vi "stepper graphics controller.vi"(4 "cursor index":i32, 6 "stepper motor state":T3, 7 "stepper graphics action":T1=enum."void", 8 "stepper graphics internal state":T2, 10 "value":dbl=1.0 format="%#_13g") -> (0 "stepper graphics internal state OUT":T2, 1 "current pos":dbl, 2 "set pos":dbl)   [LabVIEW 2018]
uses:
  stepper motor state.ctl
  stepper graphics internal state.ctl
  stepper graphics action.ctl
  2Dwindow.ctl
  slider action.ctl
  cursor action.ctl
  generate linear region.vi
  generate linear region --complex -- win cen.vi
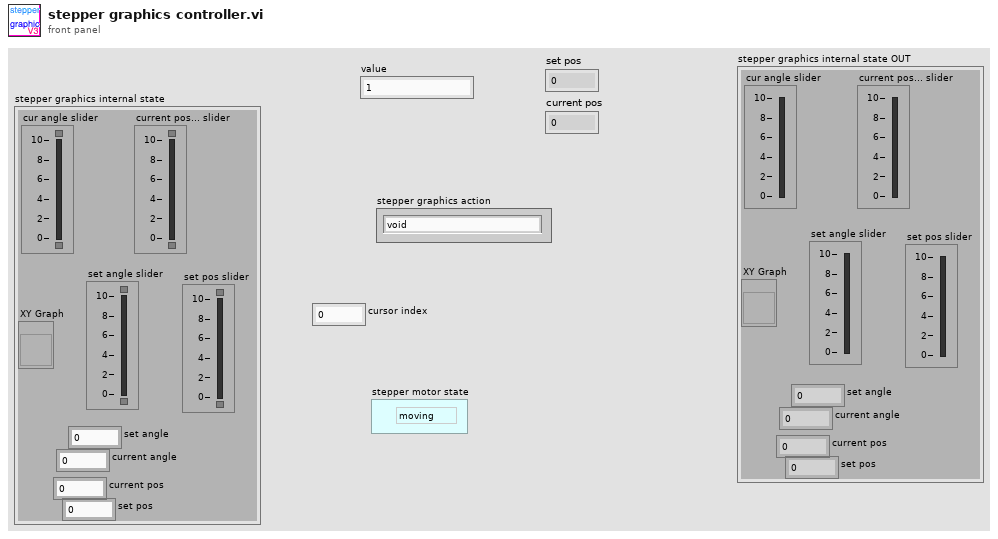
[diagram p1: front panel]
types:
  T1 = typedef "stepper graphics action.ctl" = enum16{"--update circle", "set step slider moves", "cursor moves", "current pos changed", "init", "void", "--draw current lie", "--draw set line", "--move current step slider", "--move set step slider", "--draw limit lines", "check", "--move set angle slider", "--move current angle slider", "set angle slider moves", "--move center cursor", "set set step", "set current step", "read", "--move limit-cursors", "cursor release"}
  T2 = typedef "stepper graphics internal state.ctl" = cluster{"set pos slider":refnum<vi>, "cur angle slider":refnum<vi>, "XY Graph":refnum<vi>, "set angle":dbl, "current angle":dbl, "set angle slider":refnum<vi>, "current pos... slider":refnum<vi>, "current pos":dbl, "set pos":dbl}
  T3 = typedef "stepper motor state.ctl" = enum16{"moving", "stopped"}
  T4 = typedef "2Dwindow.ctl" = cluster{"window y":dbl, "center x":dbl, "center y":dbl, "window x":dbl}
  T5 = typedef "slider action.ctl" = enum16{"check", "copy range", "set from value", "set from ratio", "set from slider", "read using other slider", "set lower limit", "set upper limit", "set lower from slider", "set upper from slider"}
  T6 = typedef "cursor action.ctl" = enum16{"range", "read", "write", "check", "zoom out", "smart zoom out", "zoom to aspect ratio 1", "zoom to win", "zoom out 20%", "zoom in 20%", "-empty", "smart zoom out&aspect", "move range left 20%", "move range right 20%", "move range up 20%", "move range down 20%", "zoom to X win", "zoom to Y win", "zoom out X", "zoom out Y", "zoom in X", "zoom in Y", "check plot scale"}
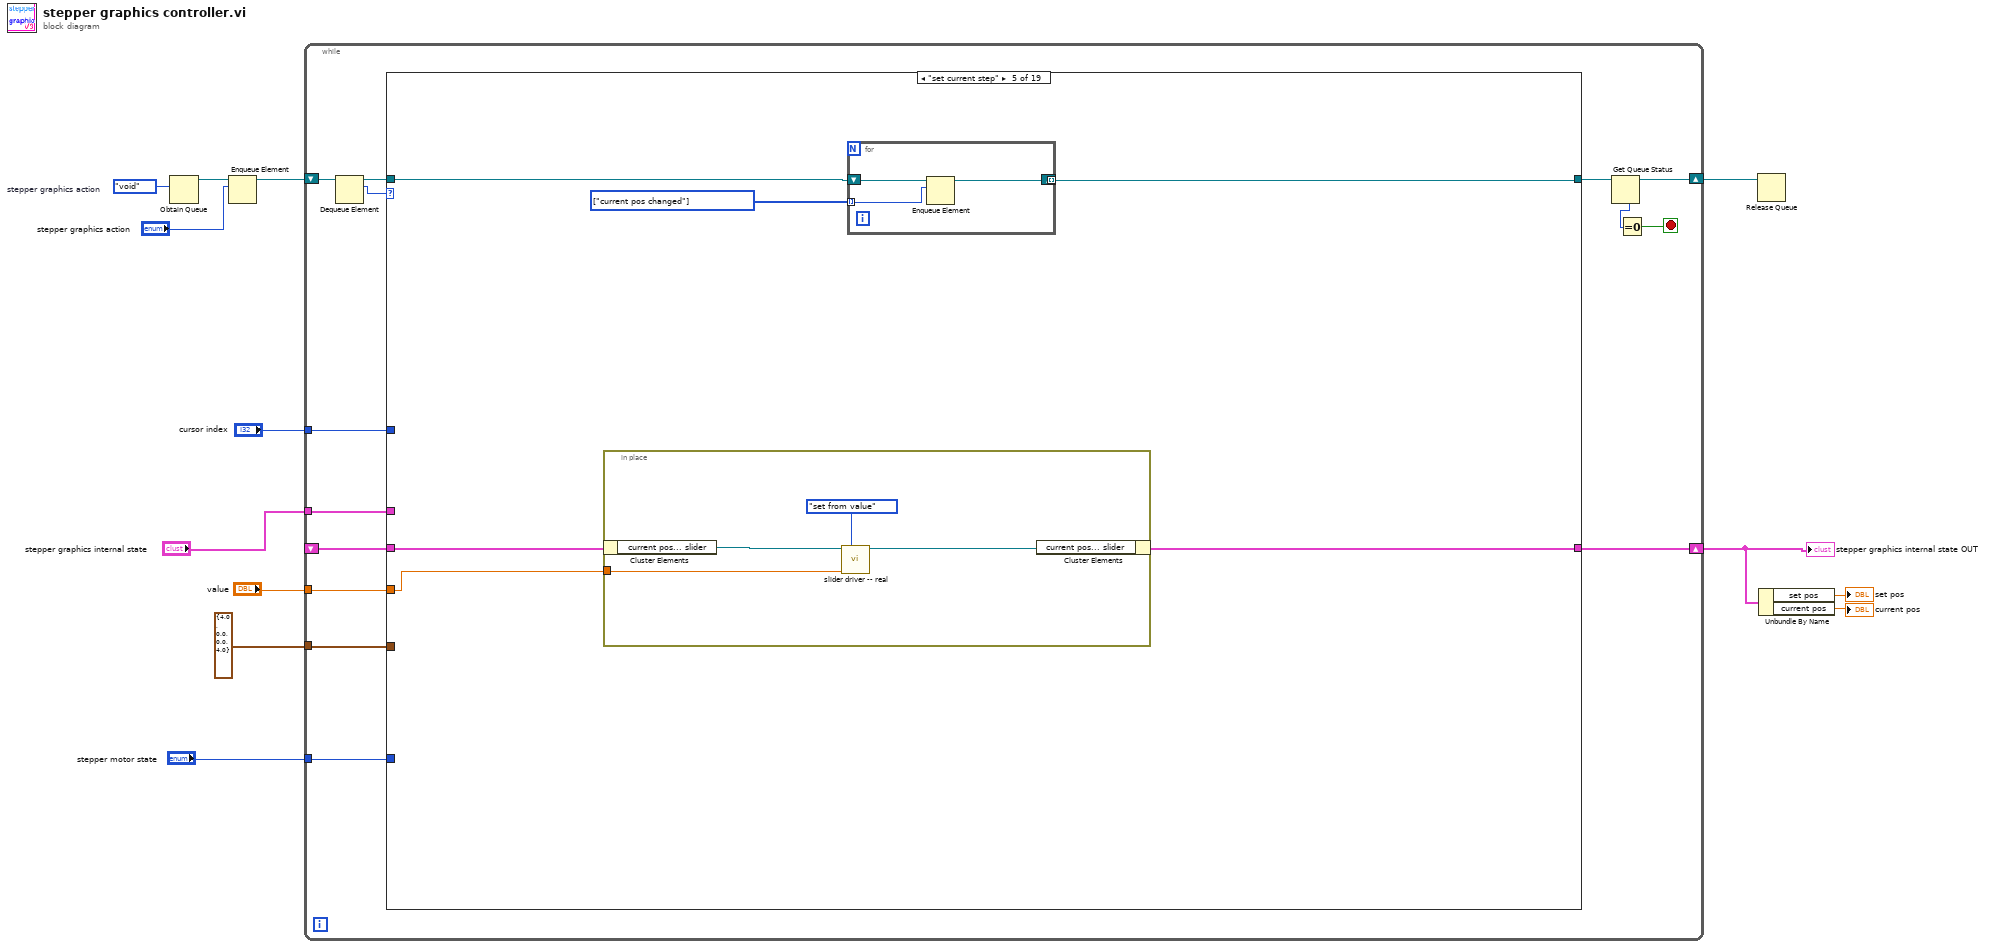
[diagram p0: block diagram]
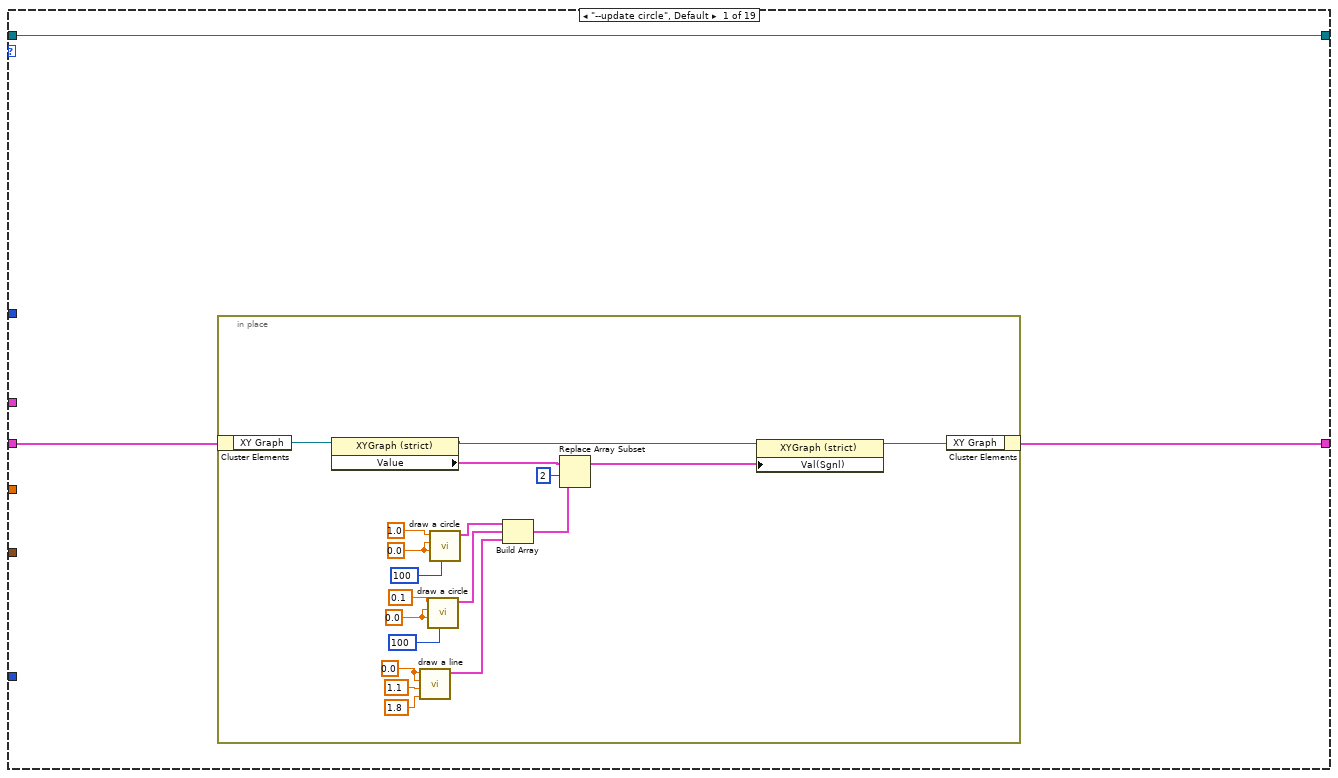
[diagram p2: hidden frame]
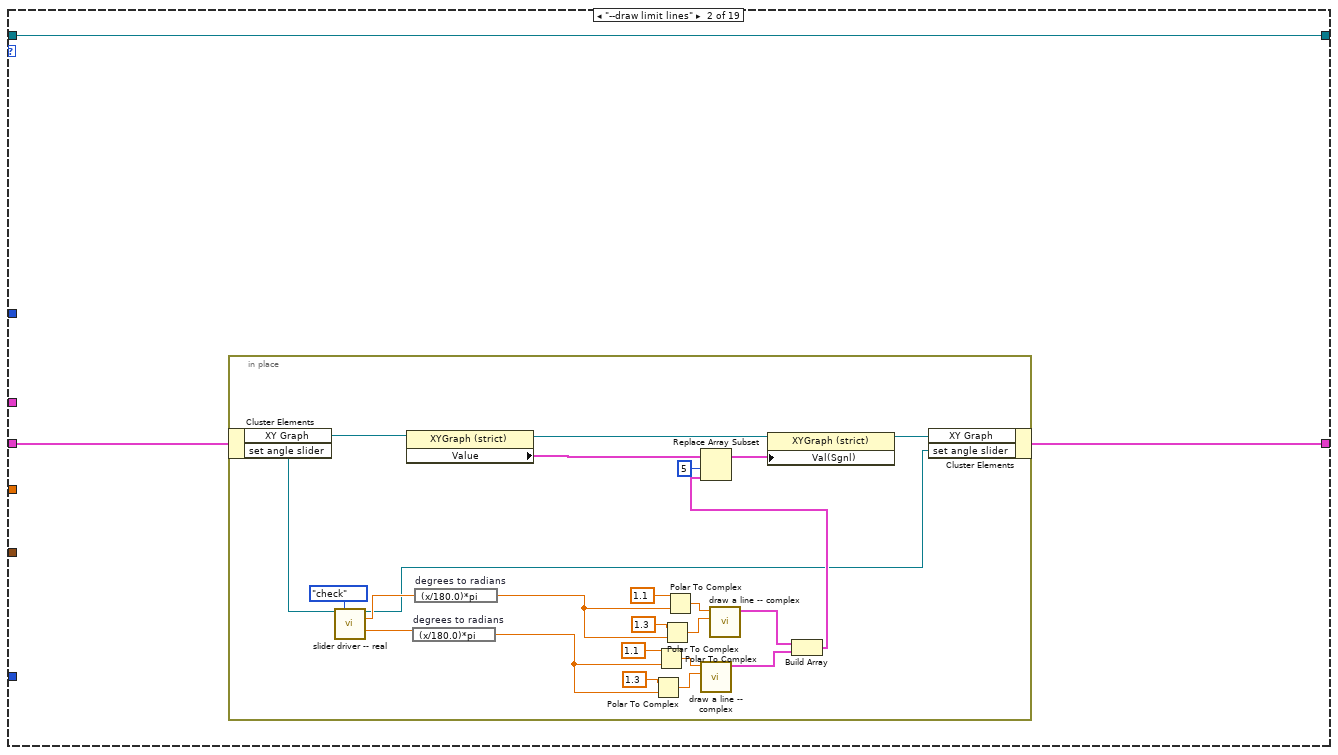
[diagram p3: hidden frame]
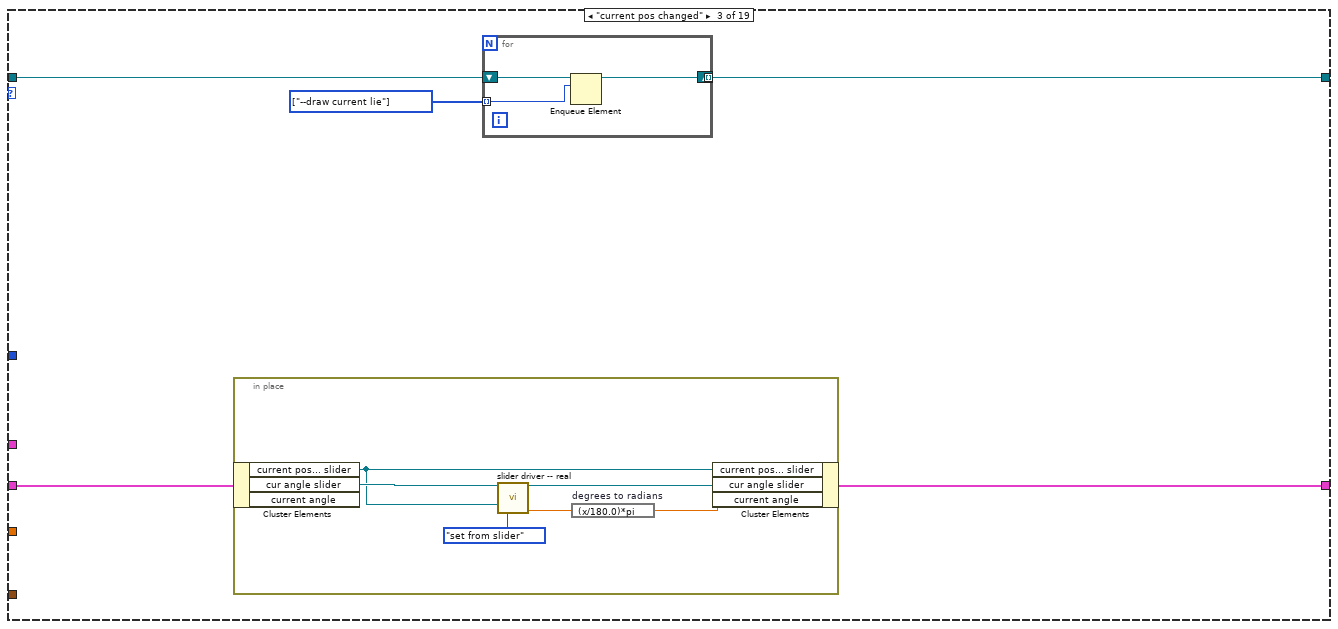
[diagram p4: hidden frame]
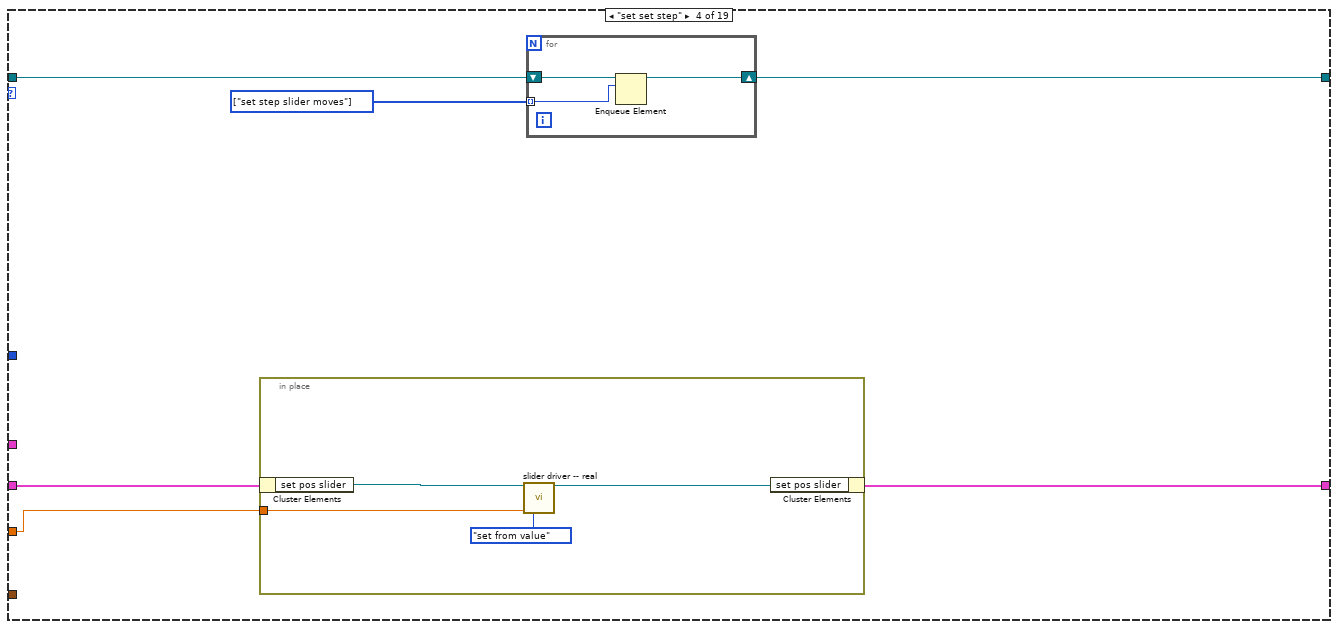
[diagram p5: hidden frame]
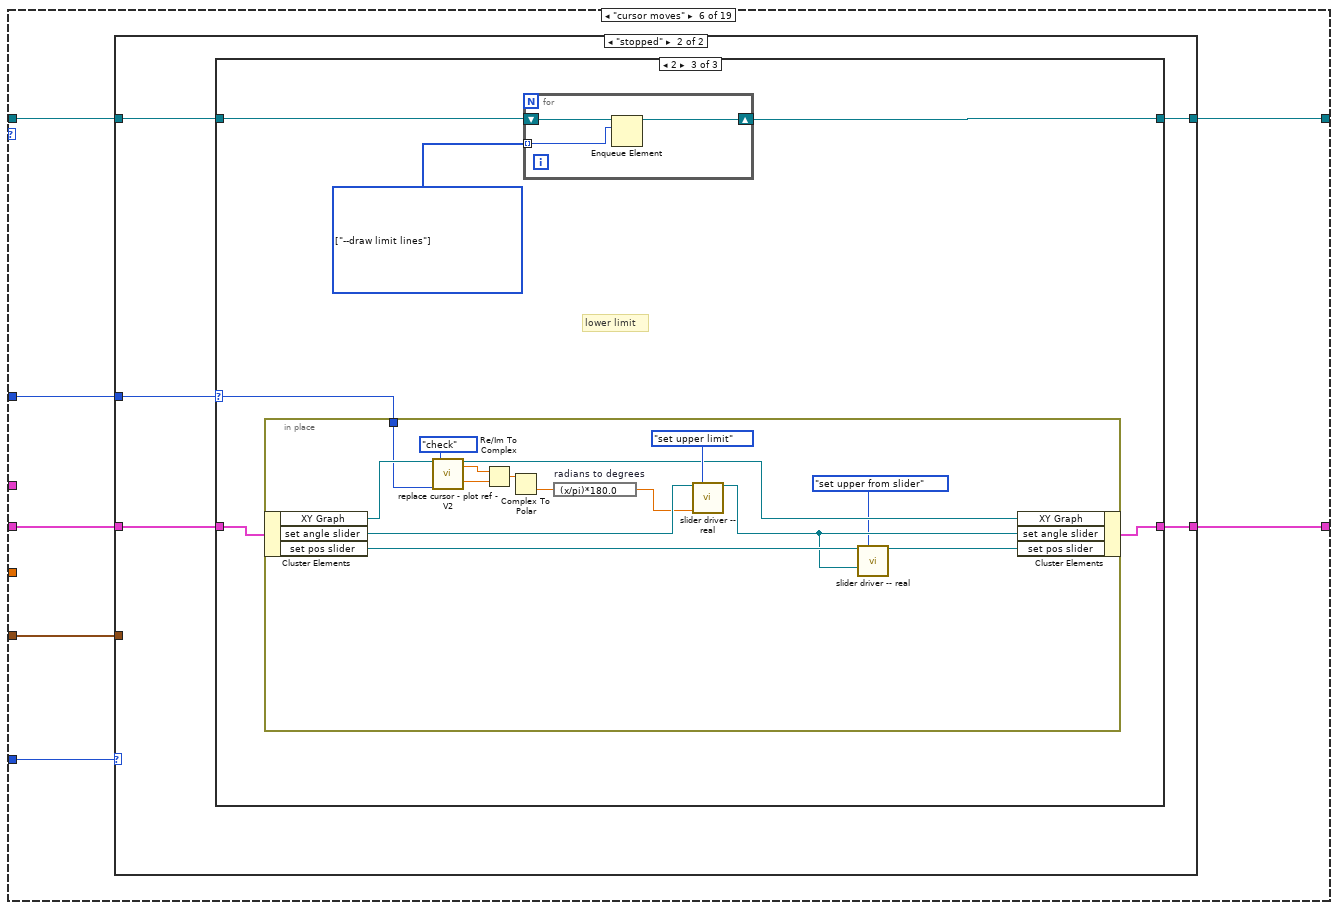
[diagram p6: hidden frame]
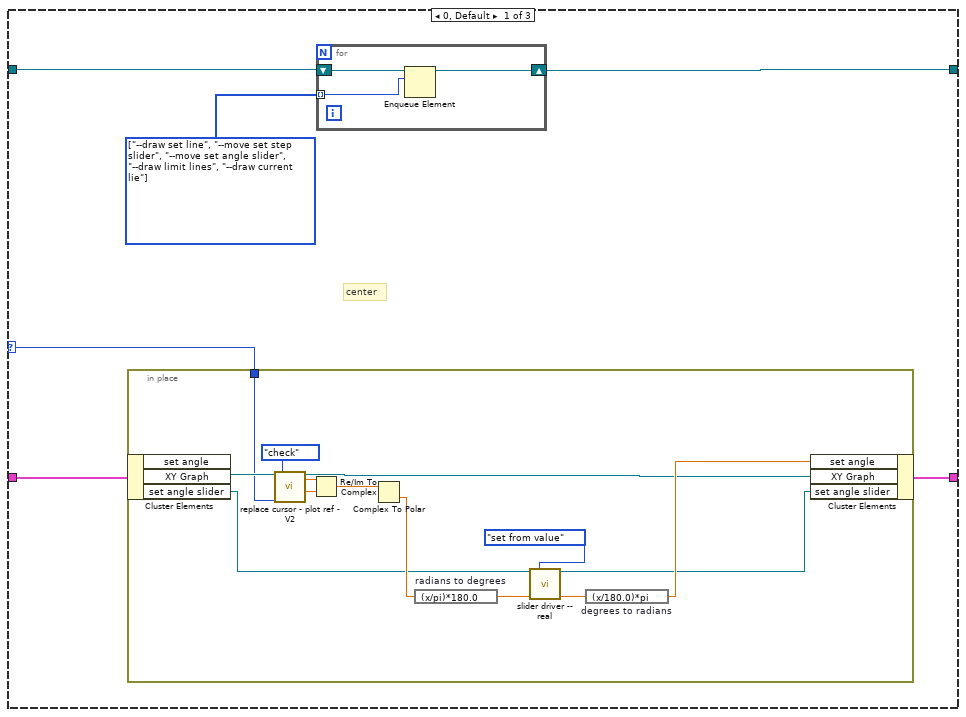
[diagram p8: hidden frame]
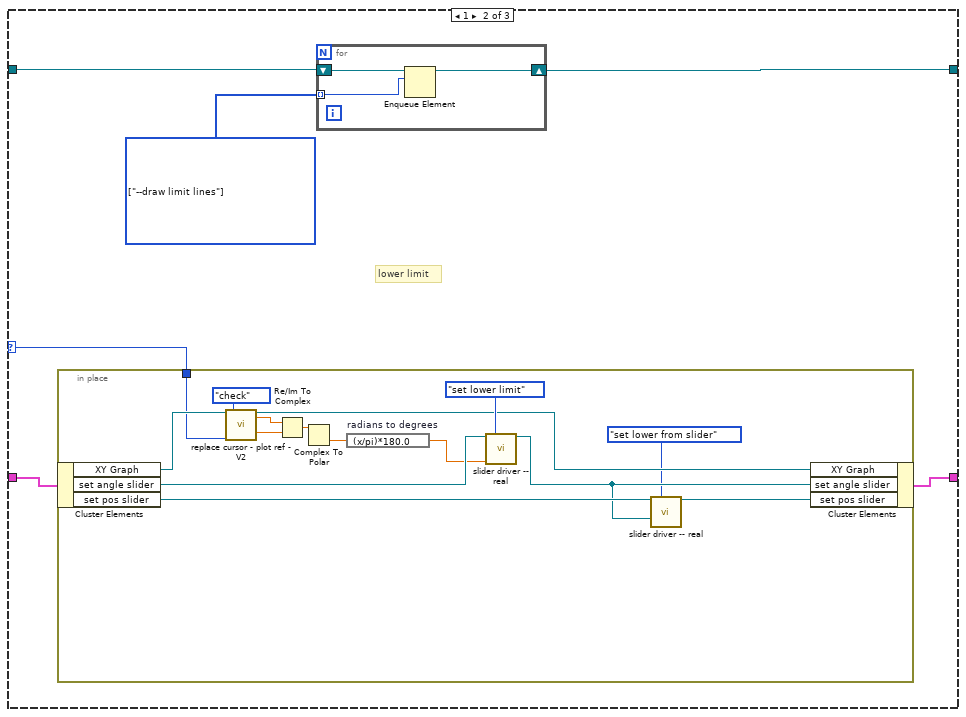
[diagram p9: hidden frame]
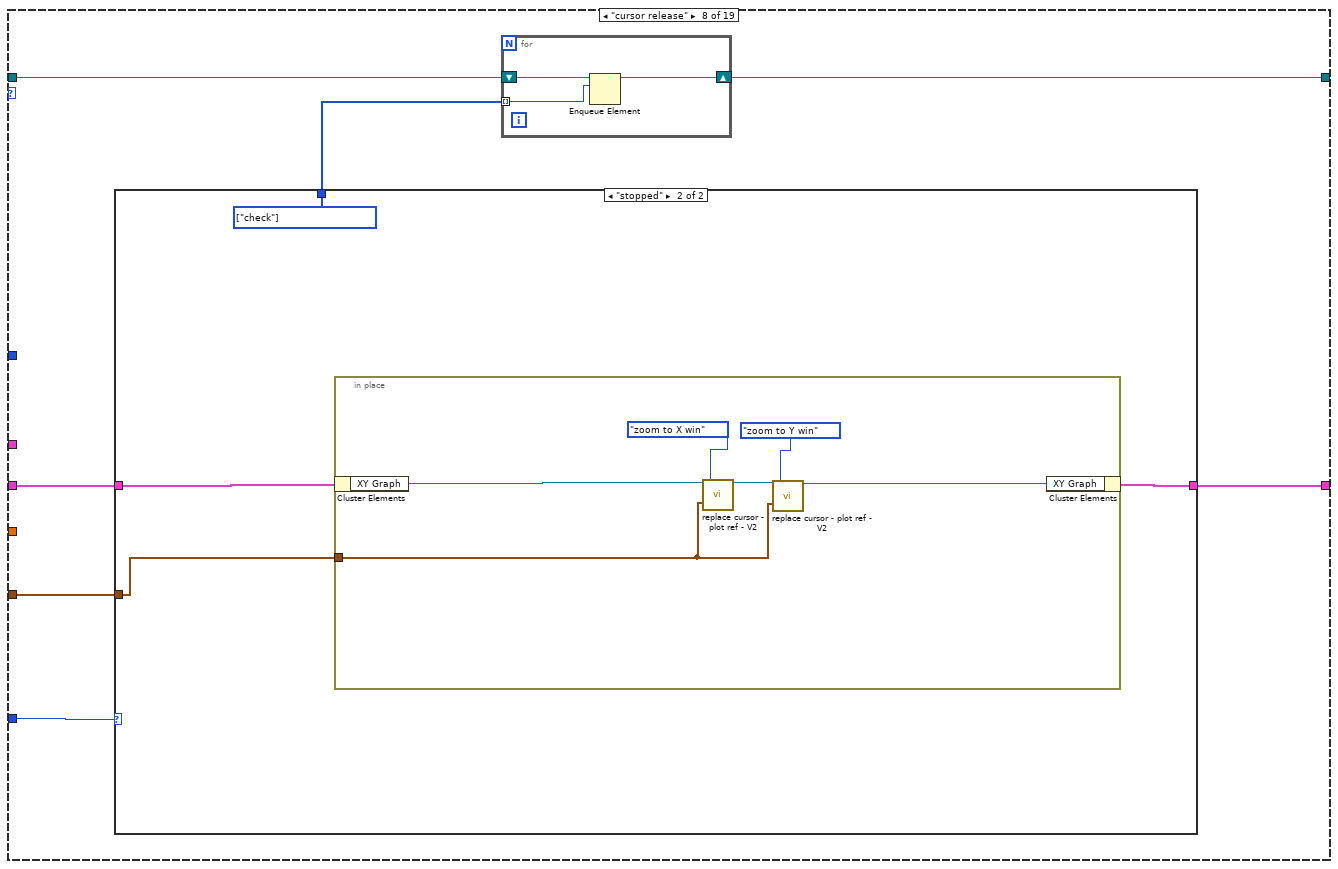
[diagram p11: hidden frame]
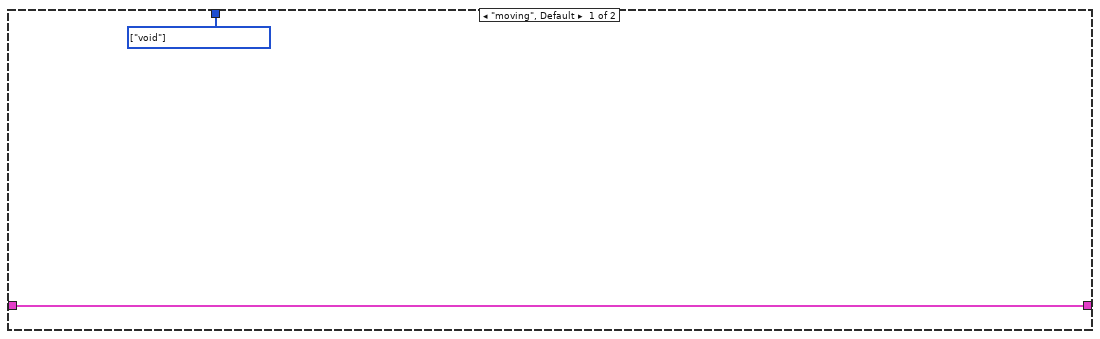
[diagram p12: hidden frame]
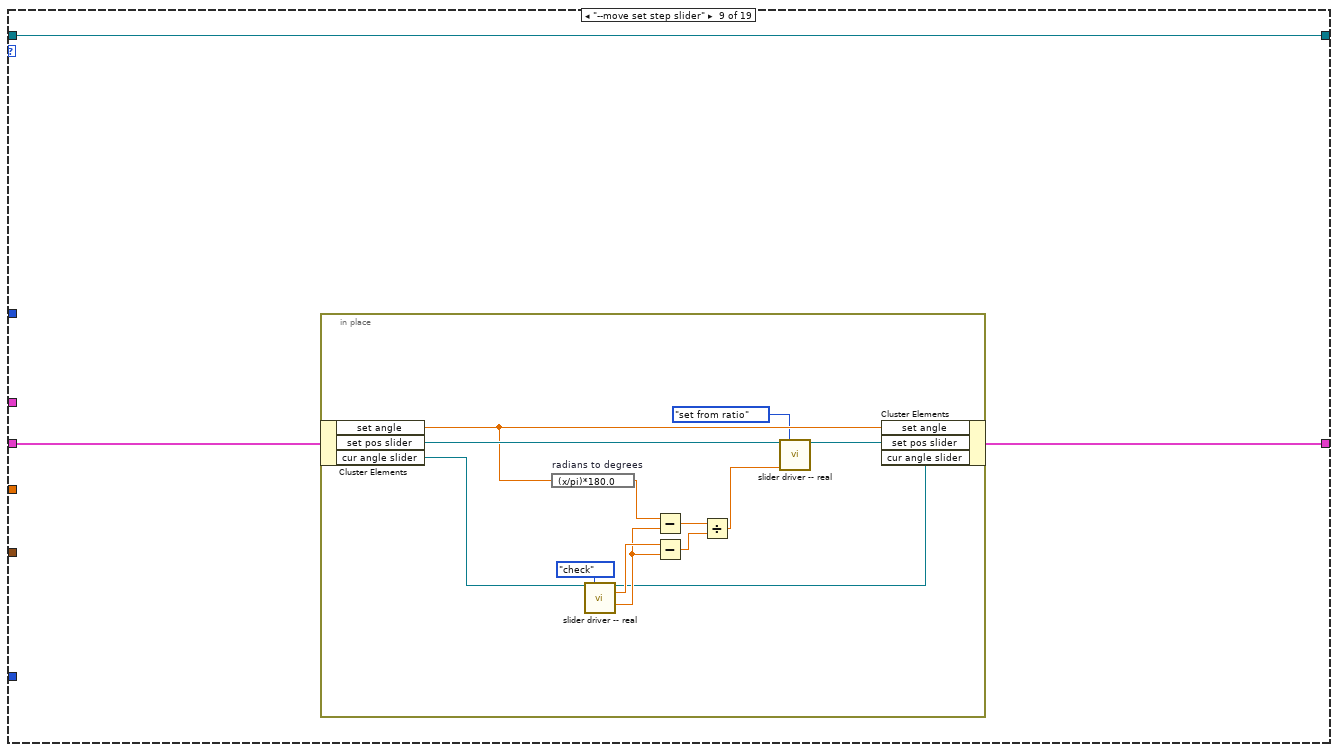
[diagram p13: hidden frame]
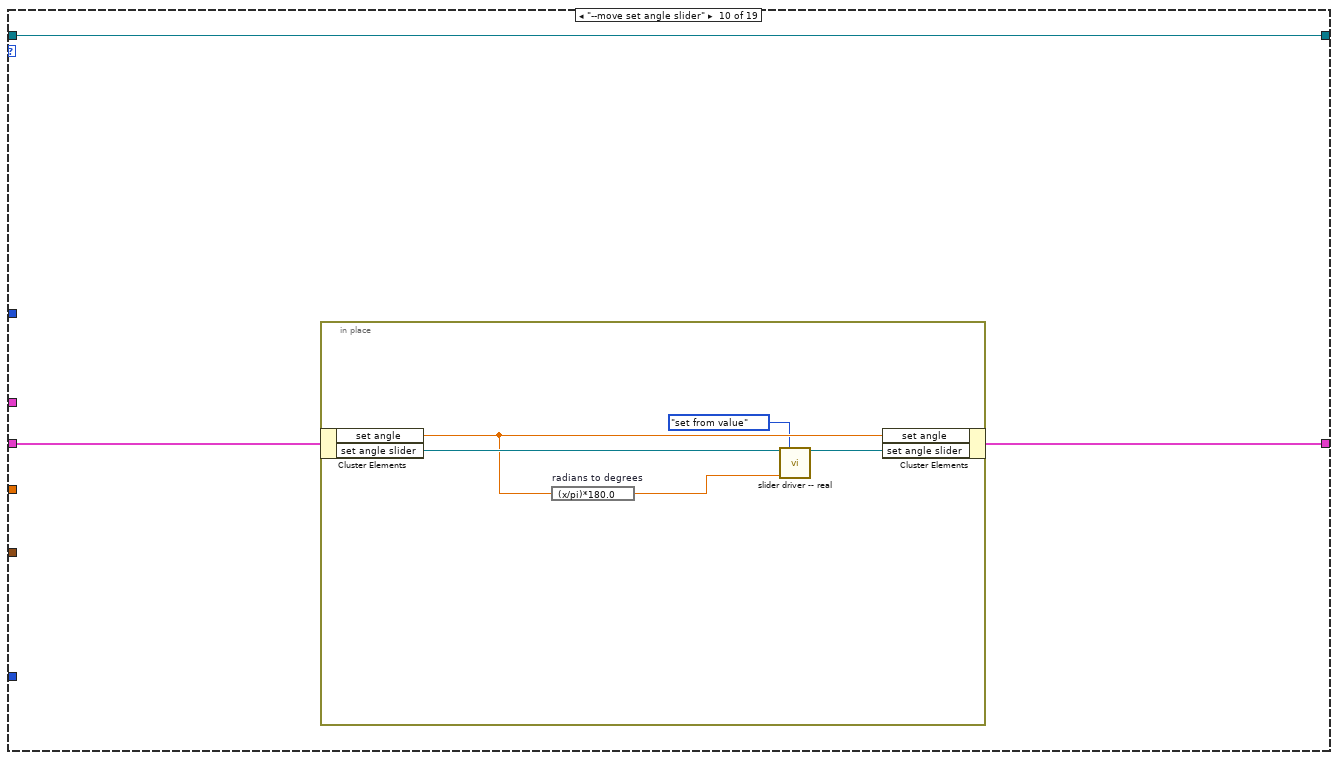
[diagram p14: hidden frame]
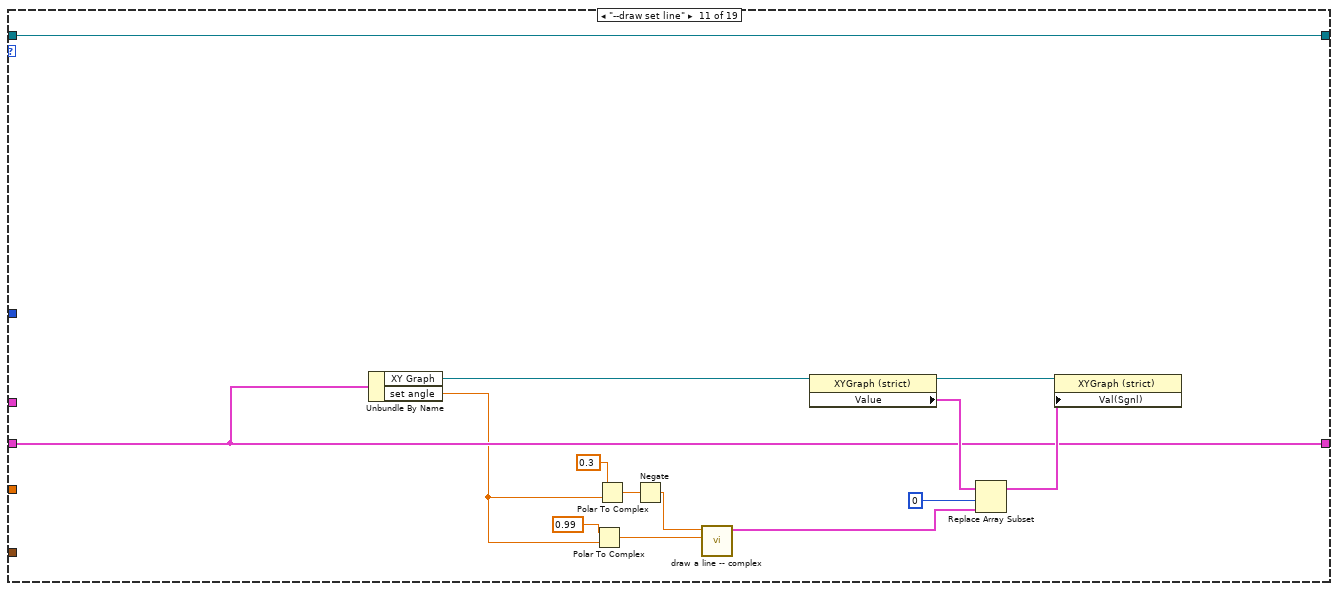
[diagram p15: hidden frame]
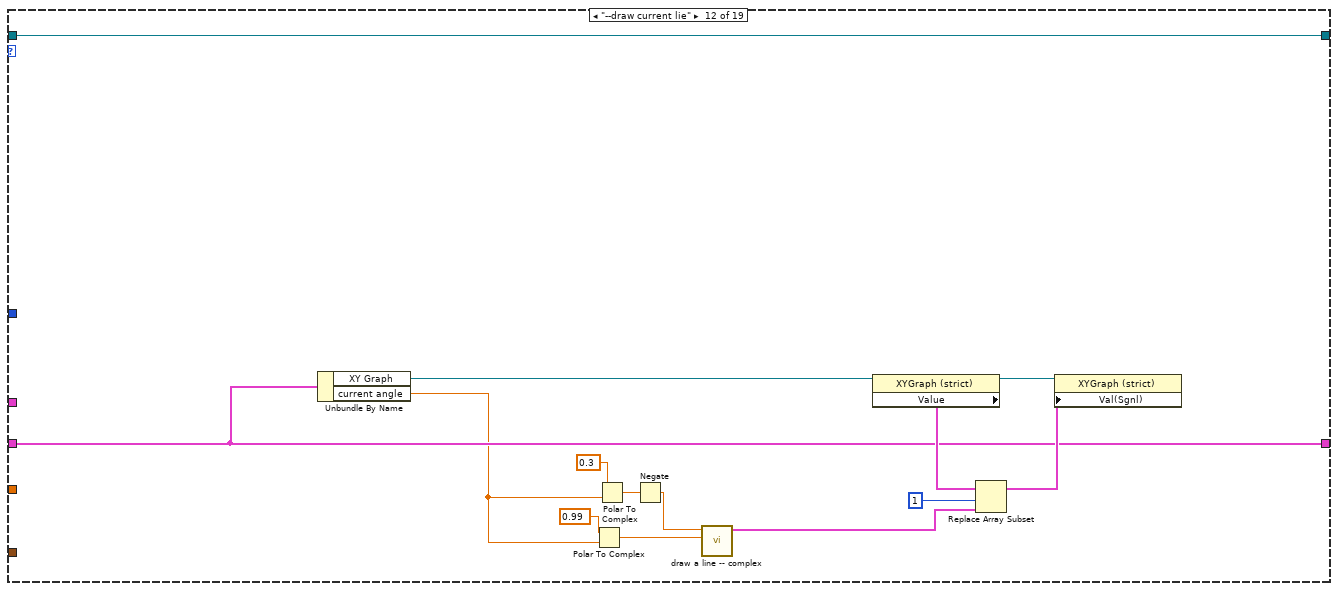
[diagram p16: hidden frame]
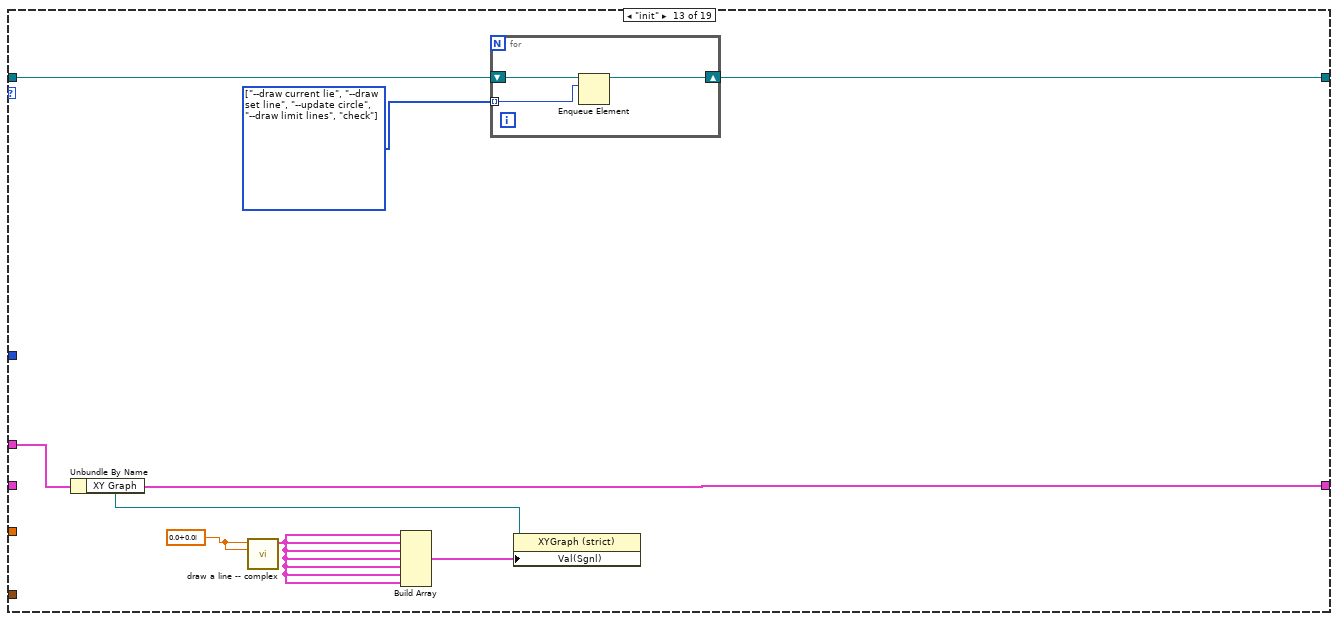
[diagram p17: hidden frame]
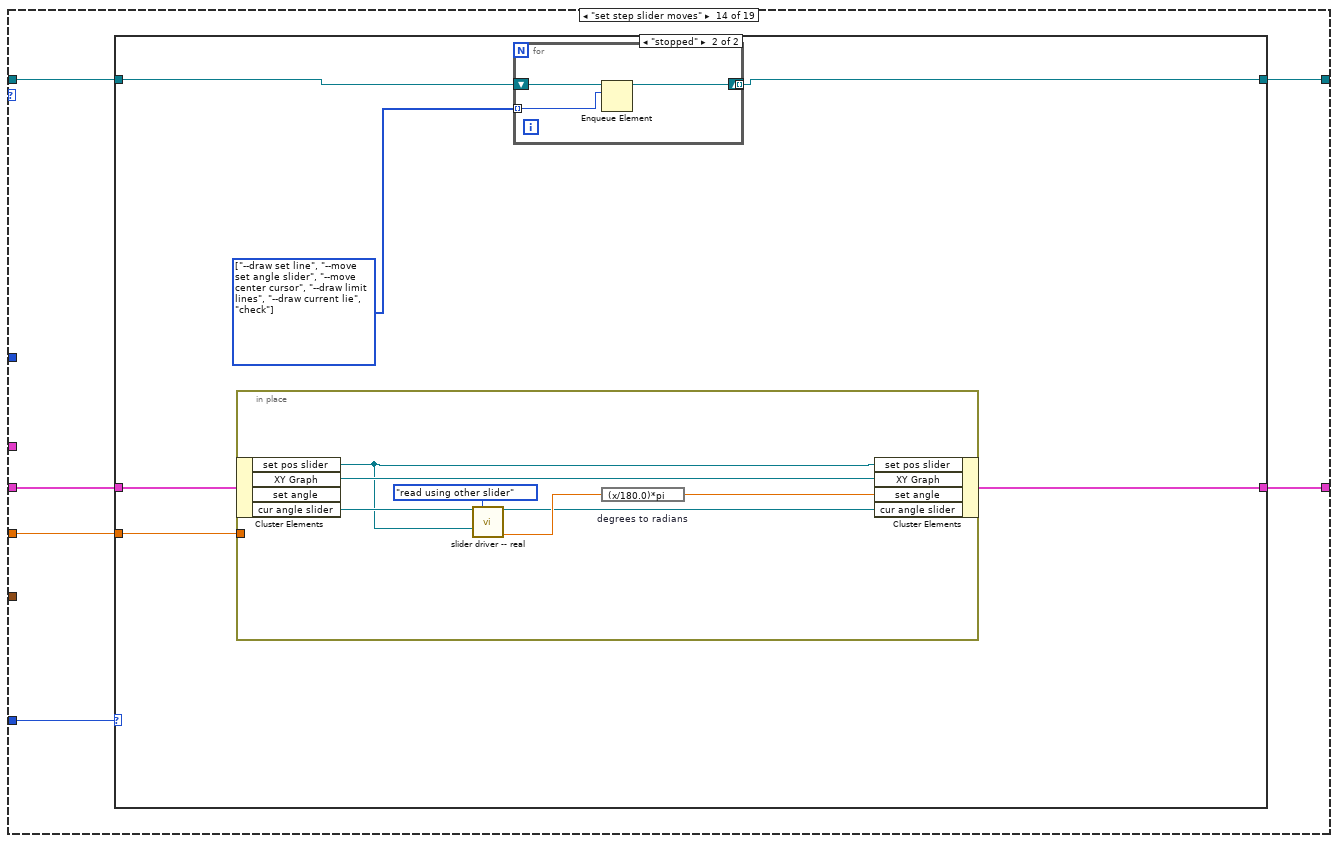
[diagram p18: hidden frame]
diagram:
  w10 = stepper_graphics_action."void"  # stepper graphics action
  n1 = Obtain Queue(element data type=w10) -> (queue out=w9:refnum<queue>)  [unwired: 4 in, 2 out]
  n2 = Enqueue Element(queue=w9, element="stepper graphics action") -> (queue out=w8:refnum<queue>)  [unwired: 2 in, 2 out]
  n3 = while {
    tunnel: "stepper motor state" -> [w27]
    tunnel: T4 {"window y"=4.0, "center x"=0.0, "center y"=0.0, "window x"=4.0} ("window IN") -> [w26]
    shift-right: [w19] -> w7
    shift-left: w8 -> [w21]
    tunnel: "stepper graphics internal state" -> [w25]
    shift-right: [w24] -> w4
    shift-left: _ -> [w23]
    tunnel: "value" -> [w22]
    tunnel: "cursor index" -> [w14]
    stop <- w16 stop-if-true
    n4 = Dequeue Element(queue=w21) -> (queue out=w15:refnum<queue>, element=w20:T1)  [unwired: 2 in, 2 out]
    n5 = case shown="\"set current step\"" w20 {
      tunnel: w27 -> [_ _ _ _ _ w123 _ w210 _ _ _ _ _ w294 w318 _ _ _ _]
      tunnel: w26 -> [_ _ _ _ _ w122 _ w209 _ _ _ _ _ _ _ _ _ w382 _]
      tunnel: w25 -> [_ _ _ _ _ _ _ _ _ _ _ _ w282 _ _ _ _ _ _]
      tunnel: [w29 w51 w80 w95 w108 w121 w202 w208 w227 w243 w253 w267 w282 w293 w317 w343 w356 w384 w416] -> w24
      tunnel: w23 -> [w30 w52 w81 w96 w109 w120 w202 w207 w228 w244 w253 w267 _ w292 w316 w342 w355 w383 w415]
      tunnel: w22 -> [_ _ _ w94 w107 _ _ _ _ _ _ _ _ w291 w315 w341 w354 _ _]
      tunnel: w15 -> [w28 w50 w78 w92 w105 w118 w203 w205 w226 w242 w250 w264 w279 w290 w314 w340 w353 w380 w414]
      tunnel: [w28 w50 w77 w91 w104 w119 w203 w204 w226 w242 w250 w264 w278 w289 w313 w340 w353 w379 w414] -> w18
      tunnel: w14 -> [_ _ _ _ _ w117 _ _ _ _ _ _ _ _ _ _ _ _ _]
      frame "--update circle", Default {
        n6 = in-place {
          w43 = 0.0 ("center x")
          w46 = 0.0 ("x0")
          w49 = 0.0 ("center x")
          n7 = in-place-cluster #1(w30) -> ("XY Graph"=w39:refnum<vi>)
          n8 = property class="XYGraph (strict)"(reference=w39) -> (reference out=w38:refnum<vi>, "Value"=w37:cluster{dbl[], dbl[]}[])  [unwired: 1 in, 1 out]
          n9 = call "draw a line.vi"("y1"=1.8 ("x0"), "y0"=1.1 ("x0"), "x1"=w46, "x0"=w46) -> ("output cluster"=w33:cluster{dbl[], dbl[]})  [unwired: 7 in]
          n10 = call "draw a circle.vi"("number of points"=100, "center Y"=w43, "center x"=w43, "radius"=0.1) -> ("output cluster"=w34:cluster{dbl[], dbl[]})  [unwired: 7 in]
          n11 = call "draw a circle.vi"("number of points"=100, "center Y"=w49, "center x"=w49, "radius"=1.0) -> ("output cluster"=w35:cluster{dbl[], dbl[]})  [unwired: 7 in]
          n12 = Build Array(w35, w34, w33) -> (w32:cluster{dbl[], dbl[]}[])
          n13 = Replace Array Subset(array=w37, new element=w32, index=2) -> (w31:cluster{dbl[], dbl[]}[])
          n14 = property class="XYGraph (strict)"(reference=w38, "Val(Sgnl)"=w31) -> (reference out=w40:refnum<vi>)  [unwired: 1 in, 1 out]
          n15 = in-place-cluster #1("XY Graph"=w40) -> (w29:T2)
        }
      }
      frame "--draw limit lines" {
        n16 = in-place {
          n17 = in-place-cluster #2(w52) -> ("XY Graph"=w75:refnum<vi>, "set angle slider"=w69:refnum<vi>)
          n18 = call "slider driver -- real.vi"("slider in"=w69, "slider action"=slider_action."check") -> ("slider out"=w53:refnum<vi>, "max"=w68:dbl, "min"=w67:dbl)  [unwired: 9 in, 2 out]
          n19 = property class="XYGraph (strict)"(reference=w75) -> (reference out=w74:refnum<vi>, "Value"=w73:cluster{dbl[], dbl[]}[])  [unwired: 1 in, 1 out]
          n20 = expression code="(x/180.0)*pi" "degrees to radians"(w67) -> (w57:dbl)
          n21 = expression code="(x/180.0)*pi" "degrees to radians"(w68) -> (w63:dbl)
          n22 = Polar To Complex(1:w57, 2:1.3 ("x")) -> (0:w59:cdb)
          n23 = Polar To Complex(1:w57, 2:1.1 ("x")) -> (0:w58:cdb)
          n24 = Polar To Complex(1:w63, 2:1.3 ("x")) -> (0:w64:cdb)
          n25 = Polar To Complex(1:w63, 2:1.1 ("x")) -> (0:w62:cdb)
          n26 = call "draw a line -- complex.vi"("x1"=w59, "x0"=w58) -> ("output cluster"=w55:cluster{dbl[], dbl[]})  [unwired: 9 in]
          n27 = call "draw a line -- complex.vi"("x1"=w64, "x0"=w62) -> ("output cluster"=w56:cluster{dbl[], dbl[]})  [unwired: 9 in]
          n28 = Build Array(w56, w55) -> (w54:cluster{dbl[], dbl[]}[])
          n29 = Replace Array Subset(array=w73, new element=w54, index=5) -> (w71:cluster{dbl[], dbl[]}[])
          n30 = property class="XYGraph (strict)"(reference=w74, "Val(Sgnl)"=w71) -> (reference out=w76:refnum<vi>)  [unwired: 1 in, 1 out]
          n31 = in-place-cluster #2("XY Graph"=w76, "set angle slider"=w53) -> (w51:T2)
        }
      }
      frame "current pos changed" {
        w79 = T1[] [enum."--draw current lie"] items=["--update circle", "set step slider moves", "cursor moves", "current pos changed", "init", "void", "--draw current lie", "--draw set line", "--move current step slider", "--move set step slider", "--draw limit lines", "check", "--move set angle slider", "--move current angle slider", "set angle slider moves", "--move center cursor", "set set step", "set current step", "read", "--move limit-cursors", "cursor release"] ("action list IN")
        n32 = in-place {
          n33 = in-place-cluster #3(w81) -> ("current pos... slider"=w85:refnum<vi>, "cur angle slider"=w90:refnum<vi>)  [unwired: 1 out]
          n34 = call "slider driver -- real.vi"("slider in"=w90, "slider action"=slider_action."set from slider", "slider from"=w85) -> ("slider out"=w87:refnum<vi>, "value OUT"=w89:dbl)  [unwired: 8 in, 3 out]
          n35 = expression code="(x/180.0)*pi" "degrees to radians"(w89) -> (w88:dbl)
          n36 = in-place-cluster #3("current pos... slider"=w85, "cur angle slider"=w87, "current angle"=w88) -> (w80:T2)
        }
        n37 = for {
          shift-right: [w82] -> w77
          shift-left: w78 -> [w84]
          tunnel: w79 -> [w83] mode=indexing
          tunnel: [w82] -> _ mode=indexing
          n38 = Enqueue Element(queue=w84, element=w83) -> (queue out=w82:refnum<queue>)  [unwired: 2 in, 2 out]
        }
      }
      frame "set set step" {
        w93 = T1[] [enum."set step slider moves"] items=["--update circle", "set step slider moves", "cursor moves", "current pos changed", "init", "void", "--draw current lie", "--draw set line", "--move current step slider", "--move set step slider", "--draw limit lines", "check", "--move set angle slider", "--move current angle slider", "set angle slider moves", "--move center cursor", "set set step", "set current step", "read", "--move limit-cursors", "cursor release"] ("action list IN")
        n39 = in-place {
          in-place-border: w94 -> [w100]
          n40 = in-place-cluster #4(w96) -> ("set pos slider"=w103:refnum<vi>)
          n41 = call "slider driver -- real.vi"("slider in"=w103, "slider action"=slider_action."set from value", "value IN"=w100) -> ("slider out"=w102:refnum<vi>)  [unwired: 8 in, 4 out]
          n42 = in-place-cluster #4("set pos slider"=w102) -> (w95:T2)
        }
        n43 = for {
          shift-right: [w97] -> w91
          shift-left: w92 -> [w99]
          tunnel: w93 -> [w98] mode=indexing
          n44 = Enqueue Element(queue=w99, element=w98) -> (queue out=w97:refnum<queue>)  [unwired: 2 in, 2 out]
        }
      }
      frame "set current step" {
        w106 = T1[] [enum."current pos changed"] items=["--update circle", "set step slider moves", "cursor moves", "current pos changed", "init", "void", "--draw current lie", "--draw set line", "--move current step slider", "--move set step slider", "--draw limit lines", "check", "--move set angle slider", "--move current angle slider", "set angle slider moves", "--move center cursor", "set set step", "set current step", "read", "--move limit-cursors", "cursor release"] ("action list IN")
        n45 = in-place {
          in-place-border: w107 -> [w113]
          n46 = in-place-cluster #5(w109) -> ("current pos... slider"=w116:refnum<vi>)
          n47 = call "slider driver -- real.vi"("slider in"=w116, "slider action"=slider_action."set from value", "value IN"=w113) -> ("slider out"=w115:refnum<vi>)  [unwired: 8 in, 4 out]
          n48 = in-place-cluster #5("current pos... slider"=w115) -> (w108:T2)
        }
        n49 = for {
          shift-right: [w110] -> w104
          shift-left: w105 -> [w112]
          tunnel: w106 -> [w111] mode=indexing
          tunnel: [w110] -> _ mode=indexing
          n50 = Enqueue Element(queue=w112, element=w111) -> (queue out=w110:refnum<queue>)  [unwired: 2 in, 2 out]
        }
      }
      frame "cursor moves" {
        n51 = case shown="\"stopped\"" w123 {
          tunnel: w122 -> [_ _]
          tunnel: [w125 w130] -> w121
          tunnel: w120 -> [w125 w129]
          tunnel: [w124 w128] -> w119
          tunnel: w118 -> [w124 w127]
          tunnel: w117 -> [_ w126]
          frame "moving", Default {
          }
          frame "stopped" {
            n52 = case shown="2" w126 {
              selector: w126 -> [w131 w154 w178]
              tunnel: [w136 w159 w183] -> w130
              tunnel: w129 -> [w135 w158 w182]
              tunnel: [w133 w156 w180] -> w128
              tunnel: w127 -> [w132 w155 w179]
              frame 0, Default {
                w134 = T1[] [enum."--draw set line", enum."--move set step slider", enum."--move set angle slider", enum."--draw limit lines", enum."--draw current lie"] items=["--update circle", "set step slider moves", "cursor moves", "current pos changed", "init", "void", "--draw current lie", "--draw set line", "--move current step slider", "--move set step slider", "--draw limit lines", "check", "--move set angle slider", "--move current angle slider", "set angle slider moves", "--move center cursor", "set set step", "set current step", "read", "--move limit-cursors", "cursor release"] ("action list IN")
                # "center"
                n53 = in-place {
                  in-place-border: w131 -> [w140]
                  n54 = in-place-cluster #6(w135) -> ("XY Graph"=w149:refnum<vi>, "set angle slider"=w147:refnum<vi>)  [unwired: 1 out]
                  n55 = call "replace cursor - plot ref - V2.vi"("Plot ref in"=w149, "cursor index"=w140, "cursor action"=cursor_action."check") -> ("Plot ref out"=w141:refnum<vi>, "read X"=w152:dbl, "read Y"=w151:dbl)  [unwired: 13 in, 1 out]
                  n56 = Re/Im To Complex(1:w151, 2:w152) -> (0:w150:cdb)
                  n57 = Complex To Polar(r * e^(i*theta)=w150) -> (theta=w148:dbl)  [unwired: 1 out]
                  n58 = expression code="(x/pi)*180.0" "radians to degrees"(w148) -> (w146:dbl)
                  n59 = call "slider driver -- real.vi"("slider in"=w147, "slider action"=slider_action."set from value", "value IN"=w146) -> ("slider out"=w142:refnum<vi>, "value OUT"=w144:dbl)  [unwired: 8 in, 3 out]
                  n60 = expression code="(x/180.0)*pi" "degrees to radians"(w144) -> (w143:dbl)
                  n61 = in-place-cluster #6("set angle"=w143, "XY Graph"=w141, "set angle slider"=w142) -> (w136:T2)
                }
                n62 = for {
                  shift-right: [w138] -> w133
                  shift-left: w132 -> [w139]
                  tunnel: w134 -> [w137] mode=indexing
                  n63 = Enqueue Element(queue=w139, element=w137) -> (queue out=w138:refnum<queue>)  [unwired: 2 in, 2 out]
                }
              }
              frame 1 {
                w157 = T1[] [enum."--draw limit lines"] items=["--update circle", "set step slider moves", "cursor moves", "current pos changed", "init", "void", "--draw current lie", "--draw set line", "--move current step slider", "--move set step slider", "--draw limit lines", "check", "--move set angle slider", "--move current angle slider", "set angle slider moves", "--move center cursor", "set set step", "set current step", "read", "--move limit-cursors", "cursor release"] ("action list IN")
                # "lower limit"
                n64 = in-place {
                  in-place-border: w154 -> [w167]
                  n65 = in-place-cluster #7(w158) -> ("XY Graph"=w173:refnum<vi>, "set angle slider"=w171:refnum<vi>, "set pos slider"=w166:refnum<vi>)
                  n66 = call "replace cursor - plot ref - V2.vi"("Plot ref in"=w173, "cursor index"=w167, "cursor action"=cursor_action."check") -> ("Plot ref out"=w168:refnum<vi>, "read X"=w176:dbl, "read Y"=w175:dbl)  [unwired: 13 in, 1 out]
                  n67 = Re/Im To Complex(1:w175, 2:w176) -> (0:w174:cdb)
                  n68 = Complex To Polar(r * e^(i*theta)=w174) -> (theta=w172:dbl)  [unwired: 1 out]
                  n69 = expression code="(x/pi)*180.0" "radians to degrees"(w172) -> (w170:dbl)
                  n70 = call "slider driver -- real.vi"("slider in"=w171, "slider action"=slider_action."set lower limit", "value IN"=w170) -> ("slider out"=w165:refnum<vi>)  [unwired: 8 in, 4 out]
                  n71 = call "slider driver -- real.vi"("slider in"=w166, "slider action"=slider_action."set lower from slider", "slider from"=w165) -> ("slider out"=w163:refnum<vi>)  [unwired: 8 in, 4 out]
                  n72 = in-place-cluster #7("XY Graph"=w168, "set angle slider"=w165, "set pos slider"=w163) -> (w159:T2)
                }
                n73 = for {
                  shift-right: [w161] -> w156
                  shift-left: w155 -> [w162]
                  tunnel: w157 -> [w160] mode=indexing
                  n74 = Enqueue Element(queue=w162, element=w160) -> (queue out=w161:refnum<queue>)  [unwired: 2 in, 2 out]
                }
              }
              frame 2 {
                w181 = T1[] [enum."--draw limit lines"] items=["--update circle", "set step slider moves", "cursor moves", "current pos changed", "init", "void", "--draw current lie", "--draw set line", "--move current step slider", "--move set step slider", "--draw limit lines", "check", "--move set angle slider", "--move current angle slider", "set angle slider moves", "--move center cursor", "set set step", "set current step", "read", "--move limit-cursors", "cursor release"] ("action list IN")
                # "lower limit"
                n75 = in-place {
                  in-place-border: w178 -> [w191]
                  n76 = in-place-cluster #8(w182) -> ("XY Graph"=w197:refnum<vi>, "set angle slider"=w195:refnum<vi>, "set pos slider"=w190:refnum<vi>)
                  n77 = call "replace cursor - plot ref - V2.vi"("Plot ref in"=w197, "cursor index"=w191, "cursor action"=cursor_action."check") -> ("Plot ref out"=w192:refnum<vi>, "read X"=w200:dbl, "read Y"=w199:dbl)  [unwired: 13 in, 1 out]
                  n78 = Re/Im To Complex(1:w199, 2:w200) -> (0:w198:cdb)
                  n79 = Complex To Polar(r * e^(i*theta)=w198) -> (theta=w196:dbl)  [unwired: 1 out]
                  n80 = expression code="(x/pi)*180.0" "radians to degrees"(w196) -> (w194:dbl)
                  n81 = call "slider driver -- real.vi"("slider in"=w195, "slider action"=slider_action."set upper limit", "value IN"=w194) -> ("slider out"=w189:refnum<vi>)  [unwired: 8 in, 4 out]
                  n82 = call "slider driver -- real.vi"("slider in"=w190, "slider action"=slider_action."set upper from slider", "slider from"=w189) -> ("slider out"=w187:refnum<vi>)  [unwired: 8 in, 4 out]
                  n83 = in-place-cluster #8("XY Graph"=w192, "set angle slider"=w189, "set pos slider"=w187) -> (w183:T2)
                }
                n84 = for {
                  shift-right: [w185] -> w180
                  shift-left: w179 -> [w186]
                  tunnel: w181 -> [w184] mode=indexing
                  n85 = Enqueue Element(queue=w186, element=w184) -> (queue out=w185:refnum<queue>)  [unwired: 2 in, 2 out]
                }
              }
            }
          }
        }
      }
      frame "void" {
      }
      frame "cursor release" {
        n86 = case shown="\"stopped\"" w210 {
          tunnel: w209 -> [_ w219]
          tunnel: [w215 w218] -> w208
          tunnel: w207 -> [w215 w217]
          tunnel: [w214 w216] -> w206
          frame "moving", Default {
            w214 = T1[] [enum."void"] items=["--update circle", "set step slider moves", "cursor moves", "current pos changed", "init", "void", "--draw current lie", "--draw set line", "--move current step slider", "--move set step slider", "--draw limit lines", "check", "--move set angle slider", "--move current angle slider", "set angle slider moves", "--move center cursor", "set set step", "set current step", "read", "--move limit-cursors", "cursor release"] ("action list IN")
          }
          frame "stopped" {
            w216 = T1[] [enum."check"] items=["--update circle", "set step slider moves", "cursor moves", "current pos changed", "init", "void", "--draw current lie", "--draw set line", "--move current step slider", "--move set step slider", "--draw limit lines", "check", "--move set angle slider", "--move current angle slider", "set angle slider moves", "--move center cursor", "set set step", "set current step", "read", "--move limit-cursors", "cursor release"] ("action list IN")
            n87 = in-place {
              in-place-border: w219 -> [w220]
              n88 = in-place-cluster #9(w217) -> ("XY Graph"=w222:refnum<vi>)
              n89 = call "replace cursor - plot ref - V2.vi"("Plot ref in"=w222, "window IN"=w220, "cursor action"=cursor_action."zoom to X win") -> ("Plot ref out"=w225:refnum<vi>)  [unwired: 13 in, 3 out]
              n90 = call "replace cursor - plot ref - V2.vi"("Plot ref in"=w225, "window IN"=w220, "cursor action"=cursor_action."zoom to Y win") -> ("Plot ref out"=w221:refnum<vi>)  [unwired: 13 in, 3 out]
              n91 = in-place-cluster #9("XY Graph"=w221) -> (w218:T2)
            }
          }
        }
        n92 = for {
          shift-right: [w212] -> w204
          shift-left: w205 -> [w213]
          tunnel: w206 -> [w211] mode=indexing
          n93 = Enqueue Element(queue=w213, element=w211) -> (queue out=w212:refnum<queue>)  [unwired: 2 in, 2 out]
        }
      }
      frame "--move set step slider" {
        n94 = in-place {
          n95 = in-place-cluster #10(w228) -> ("set angle"=w231:dbl, "set pos slider"=w233:refnum<vi>, "cur angle slider"=w234:refnum<vi>)
          n96 = expression code="(x/pi)*180.0" "radians to degrees"(w231) -> (w235:dbl)
          n97 = call "slider driver -- real.vi"("slider in"=w234, "slider action"=slider_action."check") -> ("slider out"=w230:refnum<vi>, "max"=w240:dbl, "min"=w239:dbl)  [unwired: 9 in, 2 out]
          n98 = Subtract(x=w235, y=w239) -> (x-y=w238:dbl)
          n99 = Subtract(x=w240, y=w239) -> (x-y=w237:dbl)
          n100 = Divide(x=w238, y=w237) -> (x/y=w236:dbl)
          n101 = call "slider driver -- real.vi"("slider in"=w233, "slider action"=slider_action."set from ratio", "value IN"=w236) -> ("slider out"=w232:refnum<vi>)  [unwired: 8 in, 4 out]
          n102 = in-place-cluster #10("set angle"=w231, "set pos slider"=w232, "cur angle slider"=w230) -> (w227:T2)
        }
      }
      frame "--move set angle slider" {
        n103 = in-place {
          n104 = in-place-cluster #11(w244) -> ("set angle"=w247:dbl, "set angle slider"=w249:refnum<vi>)
          n105 = expression code="(x/pi)*180.0" "radians to degrees"(w247) -> (w246:dbl)
          n106 = call "slider driver -- real.vi"("slider in"=w249, "slider action"=slider_action."set from value", "value IN"=w246) -> ("slider out"=w248:refnum<vi>)  [unwired: 8 in, 4 out]
          n107 = in-place-cluster #11("set angle"=w247, "set angle slider"=w248) -> (w243:T2)
        }
      }
      frame "--draw set line" {
        n108 = Unbundle By Name(w253) -> ("XY Graph"=w251:refnum<vi>, "set angle"=w252:dbl)
        n109 = Polar To Complex(1:w252, 2:0.99 ("x")) -> (0:w255:cdb)
        n110 = Polar To Complex(1:w252, 2:0.3 ("x")) -> (0:w257:cdb)
        n111 = Negate(x=w257) -> (-x=w256:cdb)
        n112 = call "draw a line -- complex.vi"("x1"=w255, "x0"=w256) -> ("output cluster"=w254:cluster{dbl[], dbl[]})  [unwired: 9 in]
        n113 = property class="XYGraph (strict)"(reference=w251) -> (reference out=w263:refnum<vi>, "Value"=w262:cluster{dbl[], dbl[]}[])  [unwired: 1 in, 1 out]
        n114 = Replace Array Subset(array=w262, new element=w254, index=0) -> (w261:cluster{dbl[], dbl[]}[])
        n115 = property class="XYGraph (strict)"(reference=w263, "Val(Sgnl)"=w261) -> ()  [unwired: 1 in, 2 out]
      }
      frame "--draw current lie" {
        n116 = Unbundle By Name(w267) -> ("XY Graph"=w265:refnum<vi>, "current angle"=w266:dbl)
        n117 = Polar To Complex(1:w266, 2:0.99 ("x")) -> (0:w269:cdb)
        n118 = Polar To Complex(1:w266, 2:0.3 ("x")) -> (0:w271:cdb)
        n119 = Negate(x=w271) -> (-x=w270:cdb)
        n120 = call "draw a line -- complex.vi"("x1"=w269, "x0"=w270) -> ("output cluster"=w268:cluster{dbl[], dbl[]})  [unwired: 9 in]
        n121 = property class="XYGraph (strict)"(reference=w265) -> (reference out=w277:refnum<vi>, "Value"=w276:cluster{dbl[], dbl[]}[])  [unwired: 1 in, 1 out]
        n122 = Replace Array Subset(array=w276, new element=w268, index=1) -> (w275:cluster{dbl[], dbl[]}[])
        n123 = property class="XYGraph (strict)"(reference=w277, "Val(Sgnl)"=w275) -> ()  [unwired: 1 in, 2 out]
      }
      frame "init" {
        w284 = cdb 0.0+0.0i ("x0")
        w280 = T1[] [enum."--draw current lie", enum."--draw set line", enum."--update circle", enum."--draw limit lines", enum."check"] items=["--update circle", "set step slider moves", "cursor moves", "current pos changed", "init", "void", "--draw current lie", "--draw set line", "--move current step slider", "--move set step slider", "--draw limit lines", "check", "--move set angle slider", "--move current angle slider", "set angle slider moves", "--move center cursor", "set set step", "set current step", "read", "--move limit-cursors", "cursor release"] ("action list IN")
        n124 = Unbundle By Name(w282) -> ("XY Graph"=w281:refnum<vi>)
        n125 = call "draw a line -- complex.vi"("x1"=w284, "x0"=w284) -> ("output cluster"=w283:cluster{dbl[], dbl[]})  [unwired: 9 in]
        n126 = Build Array(w283, w283, w283, w283, w283, w283, w283) -> (w285:cluster{dbl[], dbl[]}[])
        n127 = for {
          shift-right: [w286] -> w278
          shift-left: w279 -> [w288]
          tunnel: w280 -> [w287] mode=indexing
          n128 = Enqueue Element(queue=w288, element=w287) -> (queue out=w286:refnum<queue>)  [unwired: 2 in, 2 out]
        }
        n129 = property class="XYGraph (strict)"(reference=w281, "Val(Sgnl)"=w285) -> ()  [unwired: 1 in, 2 out]
      }
      frame "set step slider moves" {
        n130 = case shown="\"stopped\"" w294 {
          tunnel: w292 -> [w296 w302]
          tunnel: [w296 w301] -> w293
          tunnel: w291 -> [_ w300]
          tunnel: w290 -> [w295 w298]
          tunnel: [w295 w297] -> w289
          frame "moving", Default {
          }
          frame "stopped" {
            w299 = T1[] [enum."--draw set line", enum."--move set angle slider", enum."--move center cursor", enum."--draw limit lines", enum."--draw current lie", enum."check"] items=["--update circle", "set step slider moves", "cursor moves", "current pos changed", "init", "void", "--draw current lie", "--draw set line", "--move current step slider", "--move set step slider", "--draw limit lines", "check", "--move set angle slider", "--move current angle slider", "set angle slider moves", "--move center cursor", "set set step", "set current step", "read", "--move limit-cursors", "cursor release"] ("action list IN")
            n131 = in-place {
              in-place-border: w300 -> [_]
              n132 = in-place-cluster #12(w302) -> ("set pos slider"=w308:refnum<vi>, "XY Graph"=w309:refnum<vi>, "cur angle slider"=w311:refnum<vi>)  [unwired: 1 out]
              n133 = call "slider driver -- real.vi"("slider in"=w311, "slider action"=slider_action."read using other slider", "slider from"=w308) -> ("slider out"=w306:refnum<vi>, "value OUT"=w307:dbl)  [unwired: 8 in, 3 out]
              n134 = expression code="(x/180.0)*pi" "degrees to radians"(w307) -> (w310:dbl)
              n135 = in-place-cluster #12("set pos slider"=w308, "XY Graph"=w309, "set angle"=w310, "cur angle slider"=w306) -> (w301:T2)
            }
            n136 = for {
              shift-right: [w303] -> w297
              shift-left: w298 -> [w305]
              tunnel: w299 -> [w304] mode=indexing
              tunnel: [w303] -> _ mode=indexing
              n137 = Enqueue Element(queue=w305, element=w304) -> (queue out=w303:refnum<queue>)  [unwired: 2 in, 2 out]
            }
          }
        }
      }
      frame "set angle slider moves" {
        n138 = case shown="\"moving\", Default" w318 {
          tunnel: w316 -> [w320 w326]
          tunnel: [w320 w325] -> w317
          tunnel: w315 -> [_ w324]
          tunnel: w314 -> [w319 w322]
          tunnel: [w319 w321] -> w313
          frame "moving", Default {
          }
          frame "stopped" {
            w323 = T1[] [enum."--draw set line", enum."--move set step slider", enum."check", enum."--draw limit lines", enum."--move center cursor"] items=["--update circle", "set step slider moves", "cursor moves", "current pos changed", "init", "void", "--draw current lie", "--draw set line", "--move current step slider", "--move set step slider", "--draw limit lines", "check", "--move set angle slider", "--move current angle slider", "set angle slider moves", "--move center cursor", "set set step", "set current step", "read", "--move limit-cursors", "cursor release"] ("action list IN")
            n139 = in-place {
              in-place-border: w324 -> [w334]
              n140 = in-place-cluster #13(w326) -> ("set angle slider"=w337:refnum<vi>, "XY Graph"=w330:refnum<vi>, "set pos slider"=w336:refnum<vi>)  [unwired: 1 out]
              n141 = call "slider driver -- real.vi"("slider in"=w337, "slider action"=slider_action."check", "default"=w334) -> ("slider out"=w333:refnum<vi>, "value OUT"=w331:dbl)  [unwired: 8 in, 3 out]
              n142 = call "slider driver -- real.vi"("slider in"=w336, "slider action"=slider_action."set from slider", "slider from"=w333) -> ("slider out"=w332:refnum<vi>)  [unwired: 8 in, 4 out]
              n143 = expression code="(x/180.0)*pi" "degrees to radians"(w331) -> (w335:dbl)
              n144 = in-place-cluster #13("set angle slider"=w333, "XY Graph"=w330, "set angle"=w335, "set pos slider"=w332) -> (w325:T2)
            }
            n145 = for {
              shift-right: [w327] -> w321
              shift-left: w322 -> [w329]
              tunnel: w323 -> [w328] mode=indexing
              tunnel: [w327] -> _ mode=indexing
              n146 = Enqueue Element(queue=w329, element=w328) -> (queue out=w327:refnum<queue>)  [unwired: 2 in, 2 out]
            }
          }
        }
      }
      frame "--move center cursor" {
        n147 = in-place {
          in-place-border: w341 -> [_]
          n148 = in-place-cluster #14(w342) -> ("XY Graph"=w347:refnum<vi>, "set angle"=w345:dbl)
          n149 = Polar To Complex(1:w345, 2:1.3 ("r")) -> (0:w350:cdb)
          n150 = Complex To Re/Im(x + iy=w350) -> (x=w351:dbl, y=w352:dbl)
          n151 = call "replace cursor - plot ref - V2.vi"("Plot ref in"=w347, "new X"=w351, "new  Y"=w352, "cursor index"=0, "cursor action"=cursor_action."write") -> ("Plot ref out"=w346:refnum<vi>)  [unwired: 11 in, 3 out]
          n152 = in-place-cluster #14("XY Graph"=w346, "set angle"=w345) -> (w343:T2)
        }
      }
      frame "--move limit-cursors" {
        n153 = in-place {
          in-place-border: w354 -> [_]
          n154 = in-place-cluster #15(w355) -> ("XY Graph"=w373:refnum<vi>, "set angle slider"=w371:refnum<vi>)
          n155 = call "slider driver -- real.vi"("slider in"=w371, "slider action"=slider_action."check") -> ("slider out"=w357:refnum<vi>, "max"=w368:dbl, "min"=w369:dbl)  [unwired: 9 in, 2 out]
          n156 = expression code="(x/180.0)*pi" "degrees to radians"(w368) -> (w361:dbl)
          n157 = expression code="(x/180.0)*pi" "degrees to radians"(w369) -> (w362:dbl)
          n158 = Polar To Complex(1:w361, 2:1.5 ("r")) -> (0:w376:cdb)
          n159 = Complex To Re/Im(x + iy=w376) -> (x=w377:dbl, y=w378:dbl)
          n160 = call "replace cursor - plot ref - V2.vi"("Plot ref in"=w373, "new X"=w377, "new  Y"=w378, "cursor index"=2, "cursor action"=cursor_action."write") -> ("Plot ref out"=w359:refnum<vi>)  [unwired: 11 in, 3 out]
          n161 = Polar To Complex(1:w362, 2:1.5 ("r")) -> (0:w365:cdb)
          n162 = Complex To Re/Im(x + iy=w365) -> (x=w366:dbl, y=w367:dbl)
          n163 = call "replace cursor - plot ref - V2.vi"("Plot ref in"=w359, "new X"=w366, "new  Y"=w367, "cursor index"=1, "cursor action"=cursor_action."write") -> ("Plot ref out"=w358:refnum<vi>)  [unwired: 11 in, 3 out]
          n164 = in-place-cluster #15("XY Graph"=w358, "set angle slider"=w357) -> (w356:T2)
        }
      }
      frame "check" {
        w381 = T1[] [enum."--move center cursor", enum."--move limit-cursors"] items=["--update circle", "set step slider moves", "cursor moves", "current pos changed", "init", "void", "--draw current lie", "--draw set line", "--move current step slider", "--move set step slider", "--draw limit lines", "check", "--move set angle slider", "--move current angle slider", "set angle slider moves", "--move center cursor", "set set step", "set current step", "read", "--move limit-cursors", "cursor release"] ("action list IN")
        n165 = in-place {
          in-place-border: w382 -> [w394]
          n166 = in-place-cluster #16(w383) -> ("set pos slider"=w411:refnum<vi>, "current pos... slider"=w409:refnum<vi>, "set angle slider"=w408:refnum<vi>, "cur angle slider"=w407:refnum<vi>, "XY Graph"=w391:refnum<vi>)  [unwired: 2 out]
          n167 = call "slider driver -- real.vi"("slider in"=w411, "slider action"=slider_action."check") -> ("slider out"=w398:refnum<vi>)  [unwired: 9 in, 4 out]
          n168 = call "slider driver -- real.vi"("slider in"=w408, "slider action"=slider_action."check") -> ("slider out"=w400:refnum<vi>)  [unwired: 9 in, 4 out]
          n169 = call "slider driver -- real.vi"("slider in"=w409, "slider action"=slider_action."copy range", "slider from"=w398) -> ("slider out"=w402:refnum<vi>)  [unwired: 8 in, 4 out]
          n170 = call "slider driver -- real.vi"("slider in"=w407, "slider action"=slider_action."copy range", "slider from"=w400) -> ("slider out"=w405:refnum<vi>)  [unwired: 8 in, 4 out]
          n171 = call "slider driver -- real.vi"("slider in"=w400, "slider action"=slider_action."set from slider", "slider from"=w398) -> ("slider out"=w399:refnum<vi>, "value OUT"=w395:dbl)  [unwired: 8 in, 3 out]
          n172 = call "slider driver -- real.vi"("slider in"=w405, "slider action"=slider_action."set from slider", "slider from"=w402) -> ("slider out"=w404:refnum<vi>, "value OUT"=w389:dbl)  [unwired: 8 in, 3 out]
          n173 = expression code="(x/180.0)*pi" "degrees to radians"(w395) -> (w390:dbl)
          n174 = expression code="(x/180.0)*pi" "degrees to radians"(w389) -> (w388:dbl)
          n175 = call "replace cursor - plot ref - V2.vi"("Plot ref in"=w391, "window IN"=w394, "cursor action"=cursor_action."zoom to X win") -> ("Plot ref out"=w396:refnum<vi>)  [unwired: 13 in, 3 out]
          n176 = call "replace cursor - plot ref - V2.vi"("Plot ref in"=w396, "window IN"=w394, "cursor action"=cursor_action."zoom to Y win") -> ("Plot ref out"=w393:refnum<vi>)  [unwired: 13 in, 3 out]
          n177 = in-place-cluster #16("set pos slider"=w398, "current pos... slider"=w402, "set angle slider"=w399, "cur angle slider"=w404, "XY Graph"=w393, "set angle"=w390, "current angle"=w388) -> (w384:T2)
        }
        n178 = for {
          shift-right: [w385] -> w379
          shift-left: w380 -> [w387]
          tunnel: w381 -> [w386] mode=indexing
          tunnel: [w385] -> _ mode=indexing
          n179 = Enqueue Element(queue=w387, element=w386) -> (queue out=w385:refnum<queue>)  [unwired: 2 in, 2 out]
        }
      }
      frame "read" {
        n180 = in-place {
          n181 = in-place-cluster #17(w415) -> ("set pos slider"=w421:refnum<vi>, "current pos... slider"=w417:refnum<vi>)  [unwired: 2 out]
          n182 = call "slider driver -- real.vi"("slider in"=w421, "slider action"=slider_action."check") -> ("slider out"=w422:refnum<vi>, "value OUT"=w420:dbl)  [unwired: 9 in, 3 out]
          n183 = call "slider driver -- real.vi"("slider in"=w417, "slider action"=slider_action."check") -> ("value OUT"=w418:dbl)  [unwired: 9 in, 4 out]
          n184 = in-place-cluster #17("set pos slider"=w422, "set pos"=w420, "current pos... slider"=w417, "current pos"=w418) -> (w416:T2)
        }
      }
    }
    n185 = Get Queue Status(queue=w18) -> (queue out=w19:refnum<queue>, # elements in queue=w17:i32)  [unwired: 2 in, 6 out]
    n186 = Equal To 0?(x=w17) -> (x = 0?=w16:bool)
  }
  "stepper graphics internal state OUT" <- w4
  n187 = Release Queue(queue=w7) -> ()  [unwired: 2 in, 3 out]
  n188 = Unbundle By Name(w4) -> ("set pos"=→"set pos":dbl, "current pos"=→"current pos":dbl)
